vi "TIFFRGBA Image Begin.vi"(7 "para3":cluster{}, 8 "error in (no error)":errorcluster, 9 "para2":cluster{}, 10 "para1":cluster{}, 11 "para0":cluster{}) -> (0 "error out":errorcluster, 1 "function return":i32, 2 "para1 out":cluster{}, 3 "para0 out":cluster{}, 5 "para3 out":cluster{})   [LabVIEW 2018]
doc: "LIBTIFF_DLL_IMPEXP int TIFFRGBAImageBegin(TIFFRGBAImage*, TIFF*, int, char [1024]);\nextern int TIFFRGBAImageBegin(TIFFRGBAImage*, TIFF*, int, char [1024]);"
uses:
  libtiff3.dll
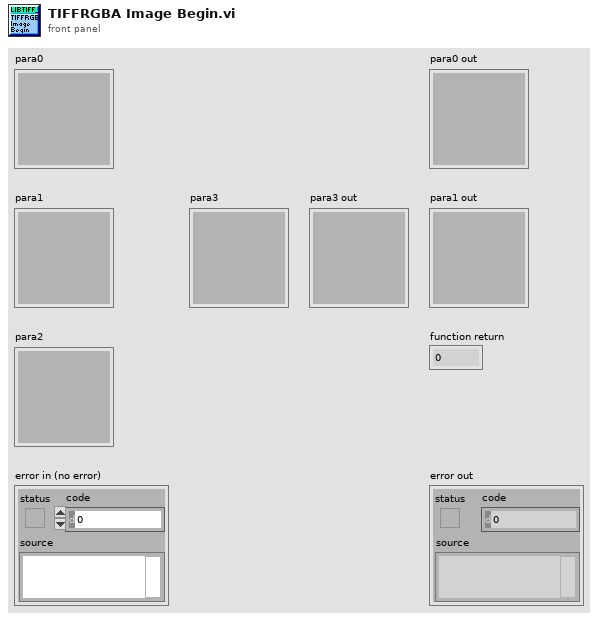
[diagram p1: front panel]
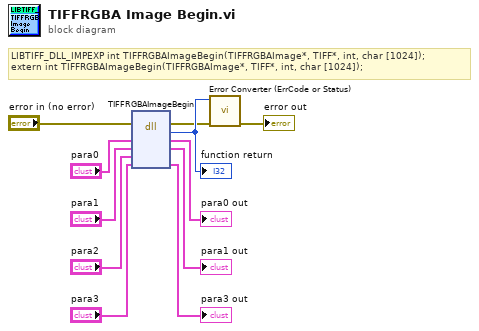
[diagram p0: block diagram]
diagram:
  # "LIBTIFF_DLL_IMPEXP\tint TIFFRGBAImageBegin(TIFFRGBAImage*, TIFF*, int, char [1024]);\nextern\tint TIFFRGBAImageBegin(TIFFRGBAImage*, TIFF*, int, char [1024]);"
  n1 = dll-call lib="C:/Users/johan/Downloads/LabVIEW software/LabVIEW software/IX-81 Software/lib/tiff/LibTiffLabview/libtiff3.*" fn="TIFFRGBAImageBegin"(error in="error in (no error)", "para0"="para0", "para1"="para1", "para2"="para2", "para3"="para3") -> (error out=w2:errorcluster, w11:i32, "para0"=→"para0 out":cluster{}, "para1"=→"para1 out":cluster{}, "para3"=→"para3 out":cluster{})  [unwired: 3 in, 1 out]
  "function return" <- w11
  n2 = call "Error Converter (ErrCode or Status).vi"("error in (no error)"=w2, "error code"=w11) -> ("error out"=→"error out":errorcluster)  [unwired: 9 in]
